vi "Sea-Level SWI Release.vi"(7 "Sea-Level SWI":T1, 8 "error in (no error)":errorcluster, 11 "Handle":i32) -> (0 "error out":errorcluster {"code" format="%.0x"})   [LabVIEW 2011]
uses:
  TypeDefs/Sea-Level SWI Adapter Info.ctl
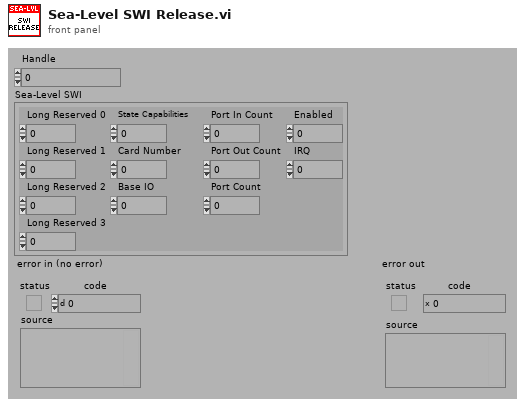
[diagram p1: front panel]
types:
  T1 = typedef "Sea-Level SWI Adapter Info.ctl" = cluster{"Long Reserved 0":i32, "Long Reserved 1":i32, "Long Reserved 2":i32, "Long Reserved 3":i32, "State Capabilities":i32, "Card Number":i16, "Base IO":i16, "Port In Count":i8, "Port Out Count":i8, "Port Count":i8, "Enabled":i8, "IRQ":i16}
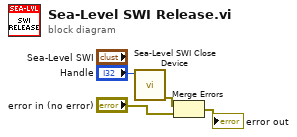
[diagram p0: block diagram]
diagram:
  n1 = call "Sea-Level SWI Close Device.vi"("Handle"="Handle") -> ("error out"=w2:errorcluster)  [unwired: 1 in, 9 out]
  n2 = Merge Errors(w2, "error in (no error)") -> (→"error out":errorcluster)
